vi "WAit Return.vi"(8 "entrée d'erreur (pas d'erreur)":errorcluster, 9 "String Wait":string="READY", 10 "VISA resource name":refnum<visa-resource-name>, 11 "Class Shielding_ Box JC-PB3044 en entrée":refnum<class "Class Shielding_ Box JC-PB3044.lvclass">) -> (0 "sortie d'erreur":errorcluster, 2 "Frame receive":string, 3 "Class Shielding_ Box JC-PB3044 en sortie":refnum<class "Class Shielding_ Box JC-PB3044.lvclass">)   [LabVIEW 2020, in "Library Instrument & Equipement.lvlib" / "Library Shielding box.lvlib" / "Class Shielding_ Box JC-PB3044.lvclass"]
uses:
  Class Shielding_ Box JC-PB3044.lvclass
  Commun VI/Library Commun.lvlib
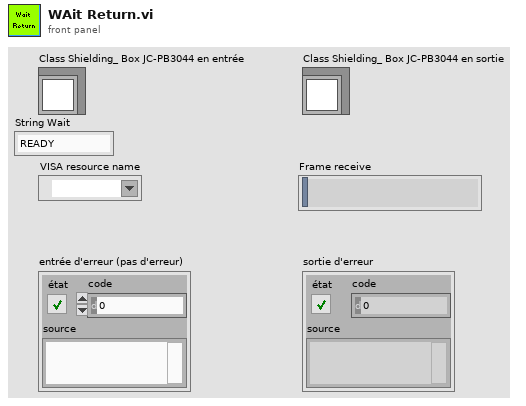
[diagram p1: front panel]
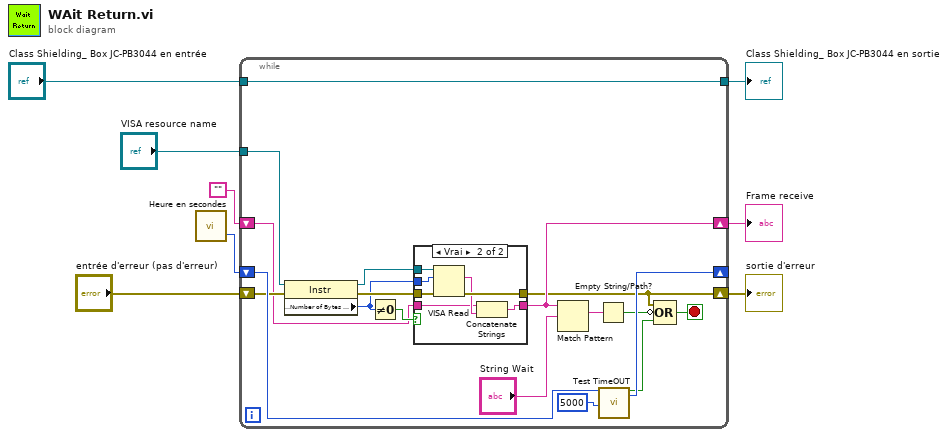
[diagram p0: block diagram]
diagram:
  n1 = call "Heure en secondes.vi"() -> ("Heure en milisecondes"=w3:u32)  [unwired: 2 in, 1 out]
  n2 = while {
    tunnel: "VISA resource name" -> [w21]
    shift-right: [w24] -> _
    shift-left: w3 -> [w26]
    shift-right: [w9] -> w5
    shift-left: "entrée d'erreur (pas d'erreur)" -> [w20]
    shift-right: [w13] -> w1
    shift-left: "" -> [w15]
    tunnel: "Class Shielding_ Box JC-PB3044 en entrée" -> [w14]
    tunnel: [w14] -> w8
    stop <- w22 stop-if-true
    n3 = property class="Instr"(reference=w21, error in=w20) -> (reference out=w18:refnum<visa-resource-name>, error out=w19:errorcluster, "Serial Settings:Number of Bytes at Serial Port"=w16:u32)
    n4 = Not Equal To 0?(x=w16) -> (x != 0?=w17:bool)
    n5 = case shown="Vrai" w17 {
      tunnel: [w28 w35] -> w9
      tunnel: w19 -> [w28 w34]
      tunnel: w18 -> [_ w33]
      tunnel: w16 -> [_ w32]
      tunnel: [w27 w30] -> w13
      tunnel: w15 -> [w27 w29]
      frame False {
      }
      frame True {
        n6 = VISA Read(VISA resource name=w33, byte count=w32, error in (no error)=w34) -> (read buffer=w31:string, error out=w35:errorcluster)  [unwired: 2 out]
        n7 = Concatenate Strings(w29, w31) -> (w30:string)
      }
    }
    n8 = Match Pattern(string=w13, regular expression="String Wait") -> (match substring=w11:string)  [unwired: 1 in, 3 out]
    n9 = Empty String/Path?(string/path=w11) -> (empty?=w10:bool)
    n10 = call "Test TimeOUT.vi"("OLD Time"=w26, "TimeOut ms"=u32 5000) -> ("Timeout ?"=w23:bool, "NEW Time"=w24:u32)  [unwired: 13 in, 3 out]
    n11 = Compound Arithmetic op=OR ("Opérateur arithmétique")(w9, invert w10, w23) -> (w22:bool)
  }
  "Class Shielding_ Box JC-PB3044 en sortie" <- w8
  "sortie d'erreur" <- w5
  "Frame receive" <- w1
